vi "DRCon.vi"() -> ()   [LabVIEW 2024]
panel:
  in  "Temperature Controller":bool
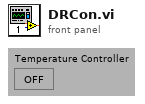
[diagram p1: front panel]
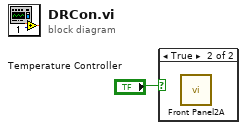
[diagram p0: block diagram]
diagram:
  n1 = case shown="True" "Temperature Controller" {
    frame False {
    }
    frame True {
      n2 = call "Front Panel2A.vi"() -> ()  [unwired: 3 in]
    }
  }
